vi "YKMW100 VF0 Relay Status.vi"(0 "VISA session":refnum<visa-resource-name>="MW100", 9 "Timeout (25000)":u32=1000, 11 "Error In":errorcluster) -> (4 "dup VISA session":refnum<visa-resource-name>, 6 "Control Relay ON (Supplying Power to Unit)":bool, 8 "DO Card Detected for Module 5":bool, 10 "Intellifaucet Relay OFF":bool, 15 "error out":errorcluster)   [LabVIEW 2016]
doc: "This VI sends the message. Then it returns the response."
panel:
  out "Read Array":string[](array[string])
  out "EN":string
  out "EA":string
  # "POWER:TRUE = OFF"
  # "FALSE = CONTACT CLOSED"
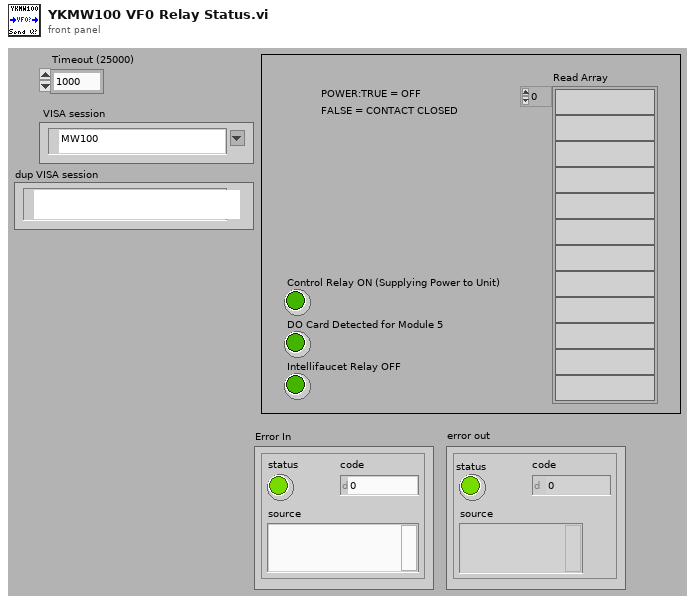
[diagram p1: front panel]
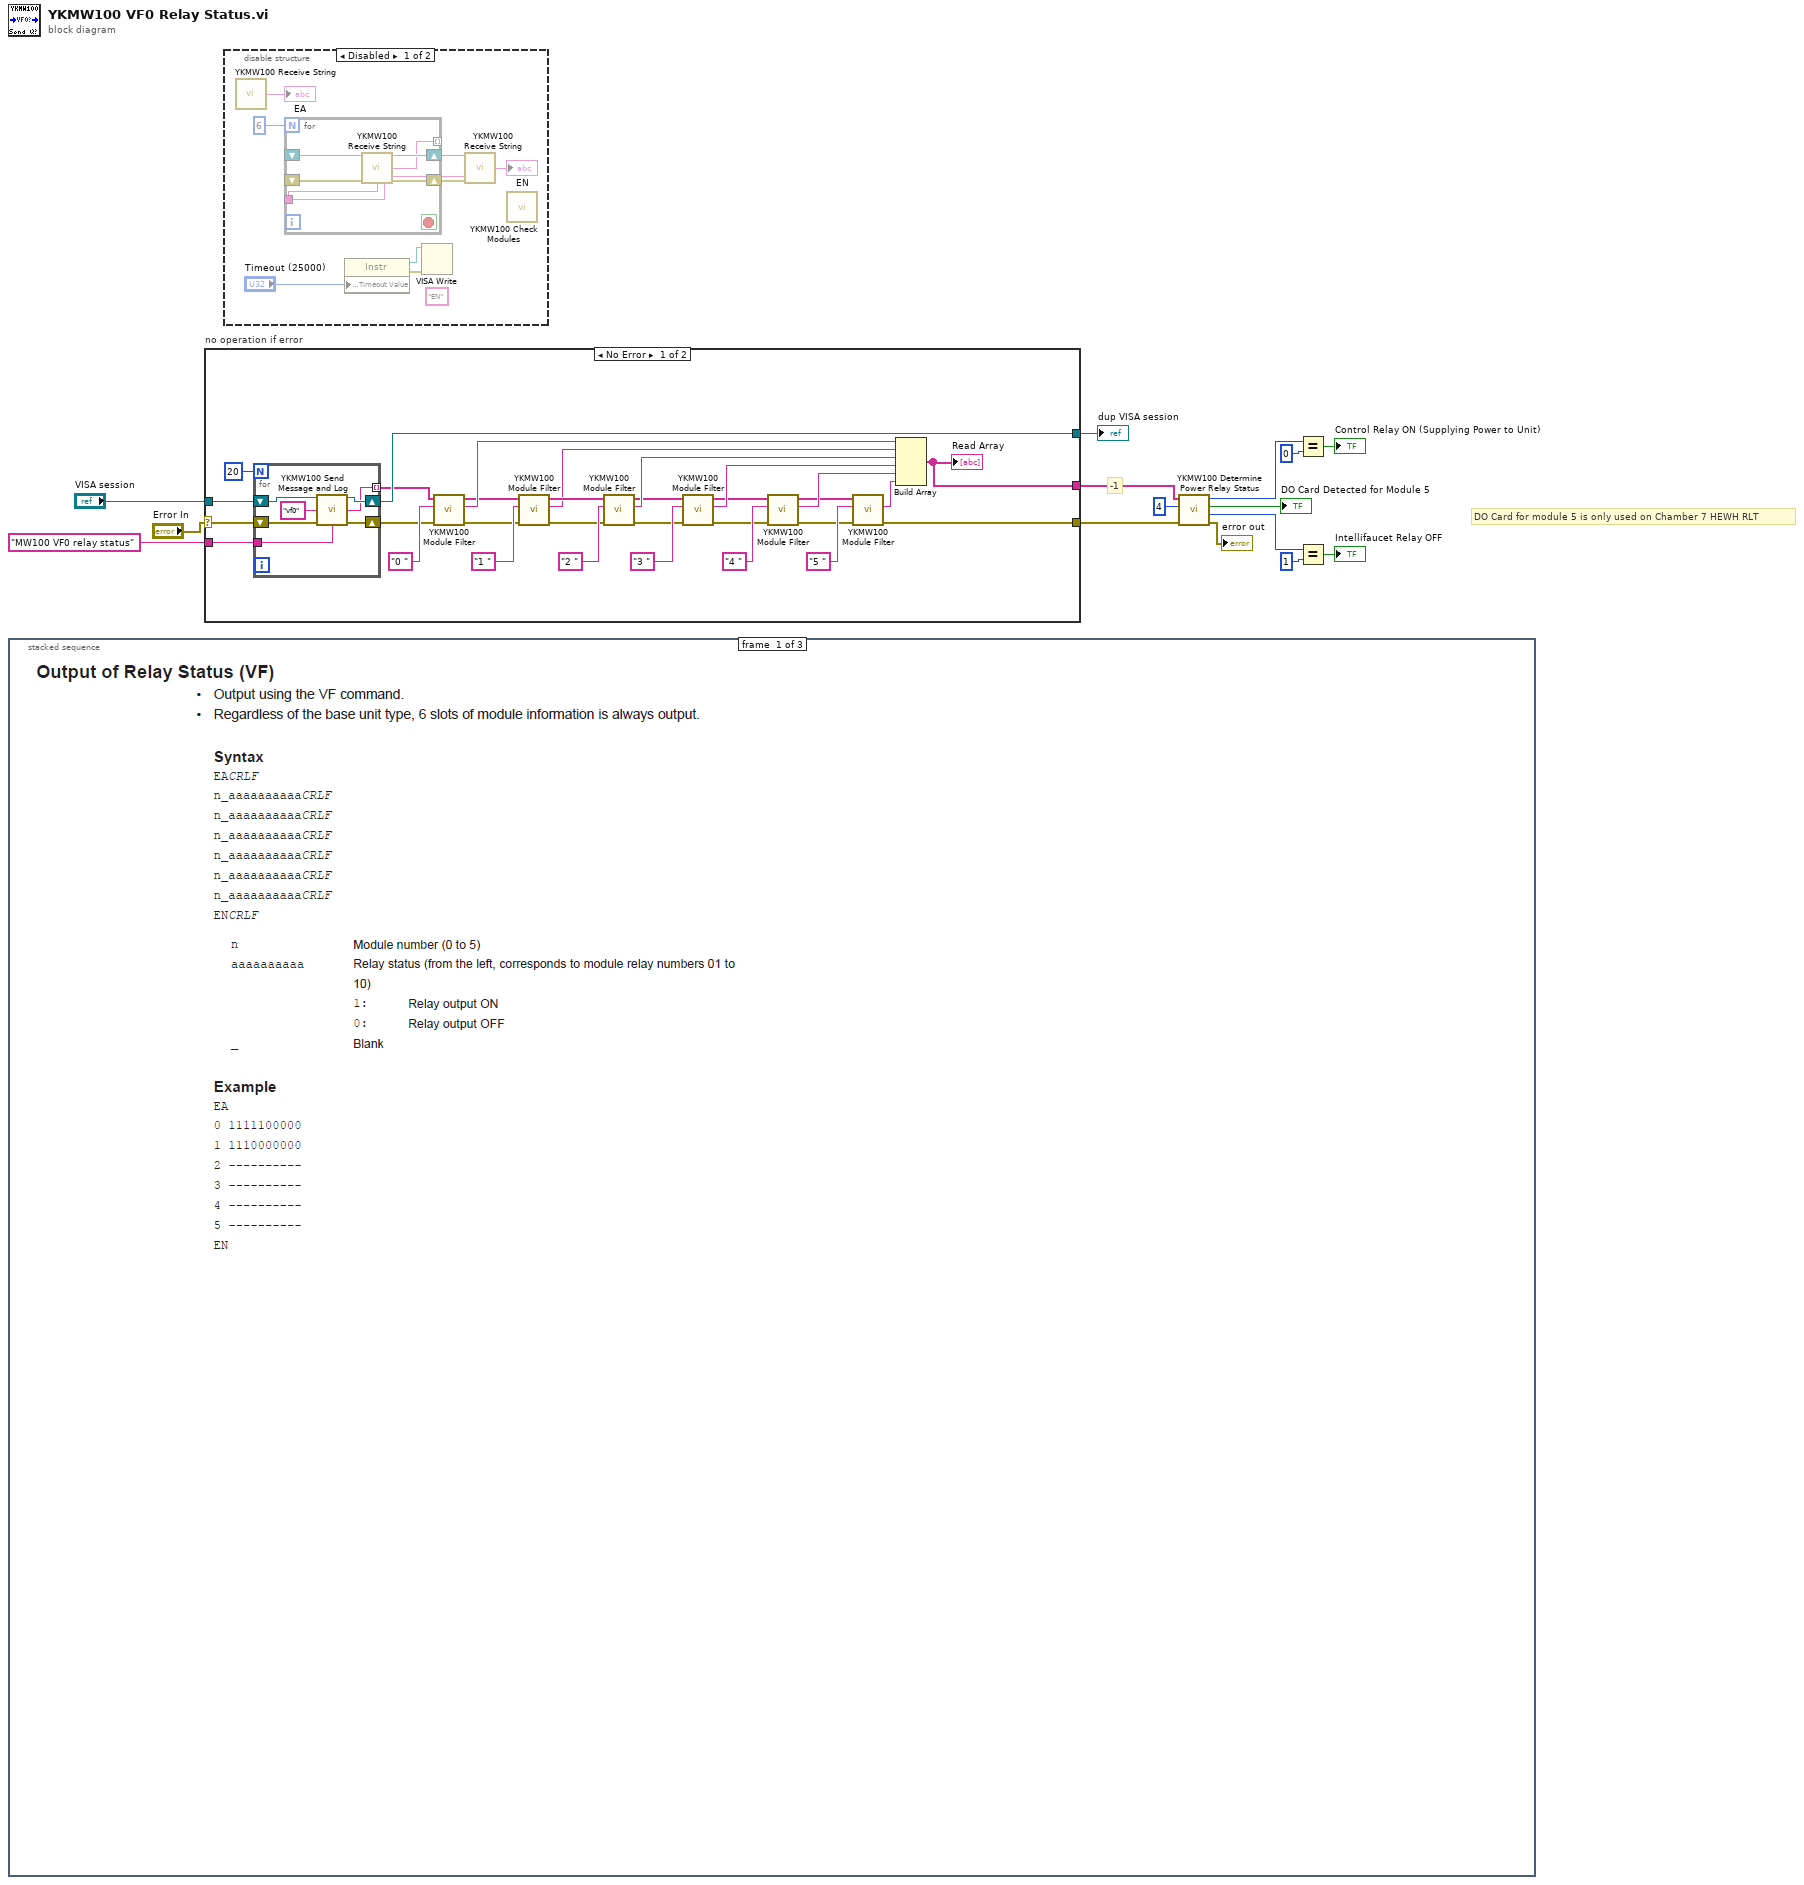
[diagram p0: block diagram]
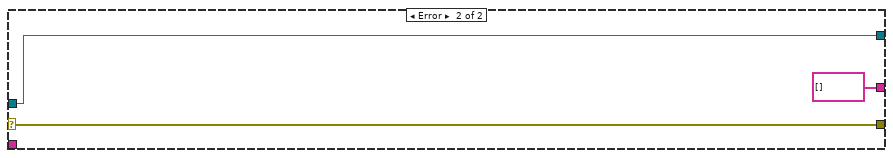
[diagram p5: hidden frame]
diagram:
  # "DO Card for module 5 is only used on Chamber 7 HEWH RLT"
  # "-1"
  n1 = stacked-sequence {
    frame #0 {
    }
    frame #1 {
      # "Used to control water valves and main power"
      # "Used for RTDs"
      # "Thermocouples"
      # "Used for Intellifaucet 4-20mA control"
      # "HEWH (Standard)"
    }
    frame #2 {
      # "The only difference in cards between RLT and standard is the additional output card in slot 5"
      # "Used to control water valves and main power"
      # "Used for RTDs"
      # "Thermocouples"
      # "Used for Intellifaucet 4-20mA control"
      # "HEWH RLT"
    }
  }
  n2 = case "no operation if error" shown="No Error" "Error In" {
    selector: "Error In" -> [w42 w54]
    tunnel: "VISA session" -> [w43 w56]
    tunnel: [w46 w56] -> w15
    tunnel: [w18 w54] -> w7
    tunnel: [w16 string[] []] -> w14
    tunnel: "MW100 VF0 relay status" ("Source (\"\")") -> [w44 _]
    frame No Error {
      n3 = for {
        N: 20 ("Numeric 4") -> [_]
        tunnel: w44 -> [w53]
        shift-right: [w49] -> w46
        shift-left: w43 -> [w51]
        shift-right: [w47] -> w19
        shift-left: w42 -> [w50]
        tunnel: [w48] -> w20 mode=indexing
        n4 = call "YKMW100 Send Message and Log.vi"("VISA session"=w51, "Send Message (\"\")"="vf0" ("Send Message (\"\")"), "error in (no error)"=w50, "Source (\"\")"=w53) -> ("dup VISA session"=w49:refnum<visa-resource-name>, "Read Buffer"=w48:string, "error out"=w47:errorcluster)  [unwired: 9 in]
      }
      n5 = call "YKMW100 Module Filter.vi"("Error In"=w19, "Select Module"="0 ", "All Data Input"=w20) -> ("Error Out"=w22:errorcluster, "Specific Point"=w37:string, "All Data Output"=w27:string[])  [unwired: 6 in]
      n6 = call "YKMW100 Module Filter.vi"("Error In"=w22, "Select Module"="1 " ("Read Buffer"), "All Data Input"=w27) -> ("Error Out"=w23:errorcluster, "Specific Point"=w17:string, "All Data Output"=w28:string[])  [unwired: 6 in]
      n7 = call "YKMW100 Module Filter.vi"("Error In"=w23, "Select Module"="2 " ("Read Buffer"), "All Data Input"=w28) -> ("Error Out"=w24:errorcluster, "Specific Point"=w38:string, "All Data Output"=w29:string[])  [unwired: 6 in]
      n8 = call "YKMW100 Module Filter.vi"("Error In"=w24, "Select Module"="3 " ("Read Buffer"), "All Data Input"=w29) -> ("Error Out"=w25:errorcluster, "Specific Point"=w39:string, "All Data Output"=w30:string[])  [unwired: 6 in]
      n9 = call "YKMW100 Module Filter.vi"("Error In"=w25, "Select Module"="4 " ("Read Buffer"), "All Data Input"=w30) -> ("Error Out"=w26:errorcluster, "Specific Point"=w40:string, "All Data Output"=w31:string[])  [unwired: 6 in]
      n10 = call "YKMW100 Module Filter.vi"("Error In"=w26, "Select Module"="5 " ("Read Buffer"), "All Data Input"=w31) -> ("Error Out"=w18:errorcluster, "Specific Point"=w41:string)  [unwired: 6 in, 1 out]
      n11 = Build Array(w37, w17, w38, w39, w40, w41) -> (w16:string[])
      "Read Array" <- w16
    }
    frame Error {
    }
  }
  "dup VISA session" <- w15
  n12 = disable-structure shown="Disabled" {
    frame Disabled {
      (unwired) "EN" ("y")
      n13 = call "YKMW100 Receive String.vi"() -> ("dup VISA session"=w70:refnum<visa-resource-name>, "Read Buffer"=→"EA":string, "Source (\"\")"=w72:string, "error out"=w71:errorcluster)  [unwired: 12 in]
      n14 = for {
        N: 6 ("Numeric 2") -> [_]
        tunnel: [w75] -> _ mode=indexing
        shift-right: [w79] -> w57
        shift-left: _ -> [w77]
        shift-right: [w78] -> w58
        shift-left: _ -> [w76]
        tunnel: [w74] -> w60
        stop <- _ stop-if-true
        n15 = call "YKMW100 Receive String.vi"("VISA session"=w77, "error in (no error)"=w76, "Source (\"\")"=w74) -> ("dup VISA session"=w79:refnum<visa-resource-name>, "Read Buffer"=w75:string, "error out"=w78:errorcluster)  [unwired: 10 in]
      }
      n16 = property class="Instr"("General Settings:Timeout Value"="Timeout (25000)") -> (reference=w64:refnum<visa-resource-name>, reference out=w65:refnum<visa-resource-name>, error in=w69:errorcluster, error out=w63:errorcluster)
      n17 = VISA Write(VISA resource name=w65, error in (no error)=w63) -> (write buffer=w62:string, VISA resource name out=w66:refnum<visa-resource-name>, error out=w67:errorcluster)  [unwired: 1 out]
      n18 = call "YKMW100 Receive String.vi"("VISA session"=w57, "error in (no error)"=w58, "Source (\"\")"=w60) -> ("Read Buffer"=→"EN":string)  [unwired: 10 in, 2 out]
      n19 = call "YKMW100 Check Modules.vi"() -> ()  [unwired: 10 in, 2 out]
    }
    frame Enabled {
    }
  }
  n20 = call "YKMW100 Determine Power Relay Status.vi"("Error In"=w7, "Module Number"=4 ("index"), "Full Module List"=w14) -> ("Error Out"=→"error out":errorcluster, "Intellifaucet Status (0=On and 1=Off)"=w1:i32, "DO Card Detected for Module 5"=→"DO Card Detected for Module 5":bool, "Relay Status (0=On and 1=Off)"=w9:i32)  [unwired: 5 in]
  n21 = Equal?(x=w9, y=0) -> (x = y?=→"Control Relay ON (Supplying Power to Unit)":bool)
  n22 = Equal?(x=w1, y=1) -> (x = y?=→"Intellifaucet Relay OFF":bool)
